vi "Cluster API String Mode.vi"(8 "error in (no error)":errorcluster, 11 "cluster api string":string="{Bool:Off;child.name:ddd}") -> (0 "error out":errorcluster, 2 "TagValue Mode":bool, 3 "Array of Strings":string[](array[string]))   [LabVIEW 2017, in "API String Arguments Support.lvlib"]
uses:
  API String Arguments Support.lvlib
  <userlib>/_NEVSTOP/Communicable State Machine(CSM)/_Shared/CSM Shared.lvlib
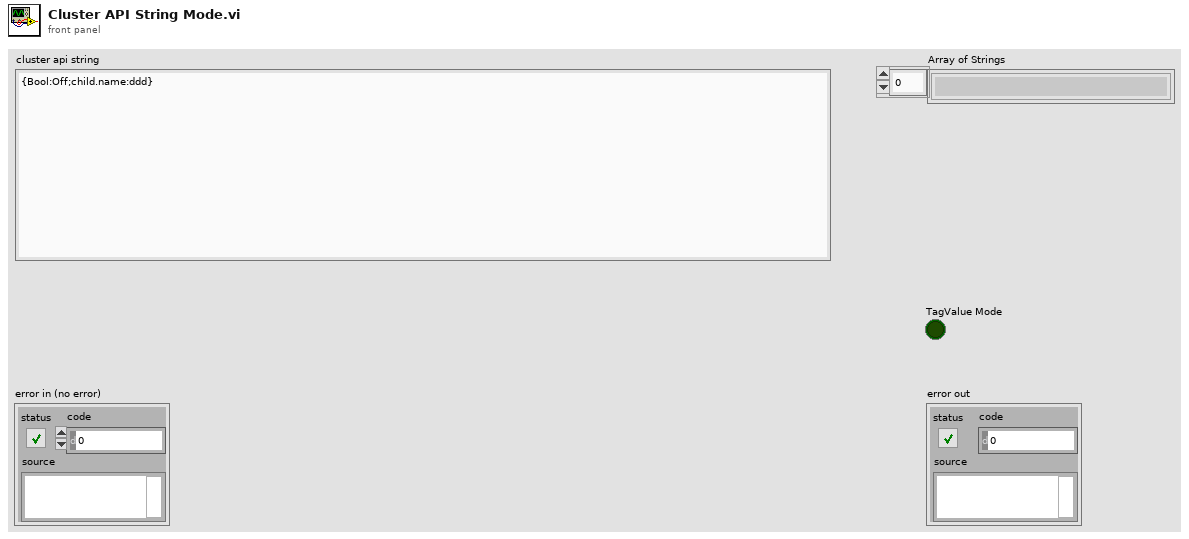
[diagram p1: front panel]
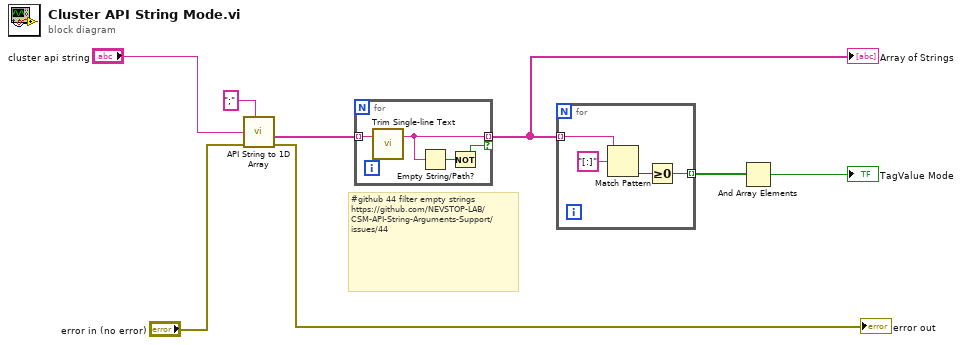
[diagram p0: block diagram]
diagram:
  # "#github 44 filter empty strings\nhttps://github.com/NEVSTOP-LAB/CSM-API-String-Arguments-Support/issues/44"
  n1 = call "API String to 1D Array.vi"("delimiter"=";" ("delimiter (Tab)"), "error in (no error)"="error in (no error)", "trimmed string in"="cluster api string") -> ("error out"=→"error out":errorcluster, "Array of Strings"=w3:string[])  [unwired: 7 in]
  n2 = for {
    tunnel: [w11] -> w2 mode=indexing if=w9
    tunnel: w3 -> [w12] mode=indexing
    n3 = call <userlib>:"Trim Single-line Text.vi"("single-line text"=w12) -> ("trimed text"=w11:string)  [unwired: 2 in]
    n4 = Empty String/Path?(string/path=w11) -> (empty?=w10:bool)
    n5 = Not(x=w10) -> (.not. x?=w9:bool)
  }
  "Array of Strings" <- w2
  n6 = for {
    tunnel: w2 -> [w15] mode=indexing
    tunnel: [w13] -> w8 mode=indexing
    n7 = Match Pattern(string=w15, regular expression="[:]") -> (offset past match=w14:i32)  [unwired: 1 in, 3 out]
    n8 = Greater Or Equal To 0?(x=w14) -> (x >= 0?=w13:bool)
  }
  n9 = And Array Elements(Boolean array=w8) -> (logical AND=→"TagValue Mode":bool)
